vi "AvgWfm.vi"(3 "ThisWfm":waveform(dbl), 4 "AvgWaveform":waveform(dbl), 5 "Numeric":i32) -> (1 "Result":waveform(dbl))   [LabVIEW 2011]
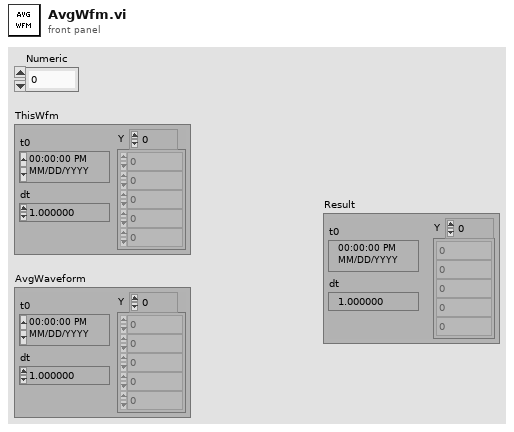
[diagram p1: front panel]
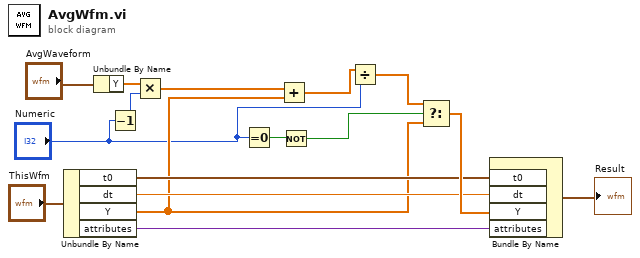
[diagram p0: block diagram]
diagram:
  n1 = Unbundle By Name("ThisWfm") -> ("t0"=w11:timestamp, "dt"=w10:dbl, "Y"=w6:dbl[], "attributes"=w9:variant)
  n2 = Unbundle By Name("AvgWaveform") -> ("Y"=w4:dbl[])
  n3 = Decrement(x="Numeric") -> (x-1=w1:i32)
  n4 = Multiply(x=w4, y=w1) -> (x*y=w3:dbl[])
  n5 = Equal To 0?(x="Numeric") -> (x = 0?=w14:bool)
  n6 = Add(x=w3, y=w6) -> (x+y=w5:dbl[])
  n7 = Not(x=w14) -> (.not. x?=w15:bool)
  n8 = Divide(x=w5, y="Numeric") -> (x/y=w7:dbl[])
  n9 = Select(t=w7, s=w15, f=w6) -> (s? t:f=w12:dbl[])
  n10 = Bundle By Name("t0"=w11, "dt"=w10, "Y"=w12, "attributes"=w9) -> (→"Result":waveform(dbl))  [unwired: 1 in]
